vi "Help.vi"(6 "reference":refnum<vi>, 8 "error in":errorcluster, 10 "SubTab":T1, 11 "Tab Control":T2) -> (0 "error out":errorcluster)   [LabVIEW 2018]
uses:
  Data Def/Main State.ctl
  Data Def/Subpanel State.ctl
  Data Def/Tips.ctl
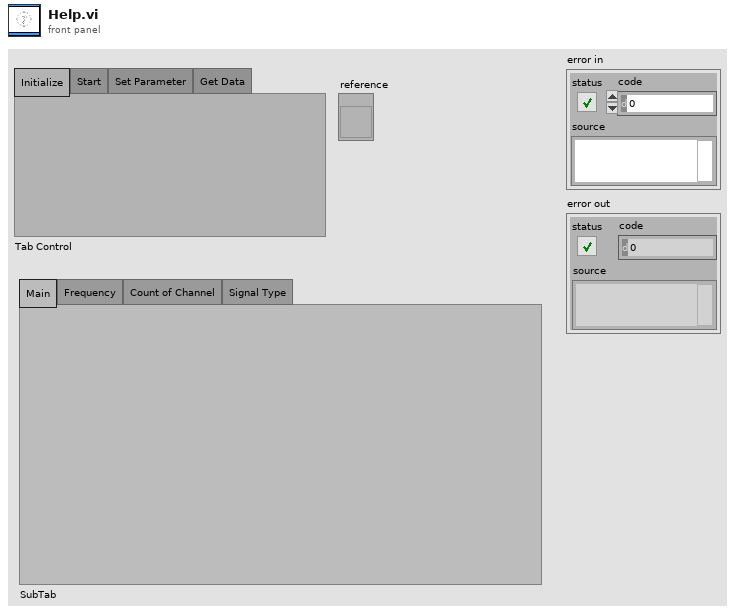
[diagram p1: front panel]
types:
  T1 = typedef "Subpanel State.ctl" = enum32{"Main", "Frequency", "Count of Channel", "Signal Type"}
  T2 = typedef "Main State.ctl" = enum32{"Initialize", "Start", "Set Parameter", "Get Data"}
  T3 = typedef "Tips.ctl" = string
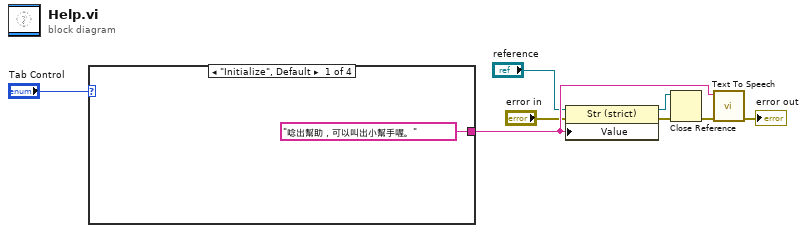
[diagram p0: block diagram]
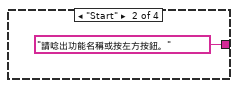
[diagram p2: hidden frame]
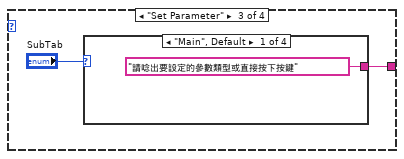
[diagram p3: hidden frame]
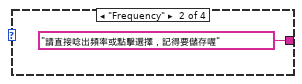
[diagram p4: hidden frame]
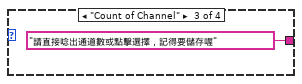
[diagram p5: hidden frame]
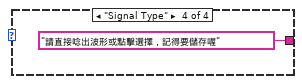
[diagram p6: hidden frame]
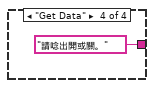
[diagram p7: hidden frame]
diagram:
  n1 = case shown="\"Initialize\", Default" "Tab Control" {
    tunnel: [T3 "唸出幫助，可以叫出小幫手喔。" ("Tips") T3 "請唸出功能名稱或按左方按鈕。" ("Tips") w11 T3 "請唸出開或關。" ("Tips")] -> w3
    frame "Initialize", Default {
    }
    frame "Start" {
    }
    frame "Set Parameter" {
      n2 = case shown="\"Main\", Default" "SubTab" {
        tunnel: ["請唸出要設定的參數類型或直接按下按鍵" "請直接唸出頻率或點擊選擇，記得要儲存喔" "請直接唸出通道數或點擊選擇，記得要儲存喔" "請直接唸出波形或點擊選擇，記得要儲存喔"] -> w11
        frame "Main", Default {
        }
        frame "Frequency" {
        }
        frame "Count of Channel" {
        }
        frame "Signal Type" {
        }
      }
    }
    frame "Get Data" {
    }
  }
  n3 = property class="Str (strict)"(reference="reference", error in="error in", "Value"=w3) -> (reference out=w5:refnum<vi>, error out=w6:errorcluster)
  n4 = Close Reference(reference=w5, error in (no error)=w6) -> (error out=w4:errorcluster)
  n5 = call "Text To Speech.vi"("error in (no error)"=w4, "textToSpeak"=w3) -> ("error out"=→"error out":errorcluster)  [unwired: 9 in]
